vi "Query Heater Status.vi"(8 "error in (no error)":errorcluster, 10 "Output (0:Sample Heater)":u16(ring) items=["Sample Heater", "Warm-up Heater (Output 1)"], 11 "VISA resource name":refnum<visa-resource-name>) -> (0 "error out":errorcluster, 2 "Heater Status":u16(ring) items=["No Error (0)", "Heater Open Error (1)", "Heater Short Error (2)", "Voltage Compliance (3)"], 3 "VISA resource name out":refnum<visa-resource-name>)   [LabVIEW 2015, in "Lake Shore 372.lvlib"]
doc: "Queries if there is a heater open error.\n\nNote:\nThis only applies to sample heater and output 1 (warm-up heater)."
uses:
  <instrlib>/Lake Shore 372/Lake Shore 372.lvlib
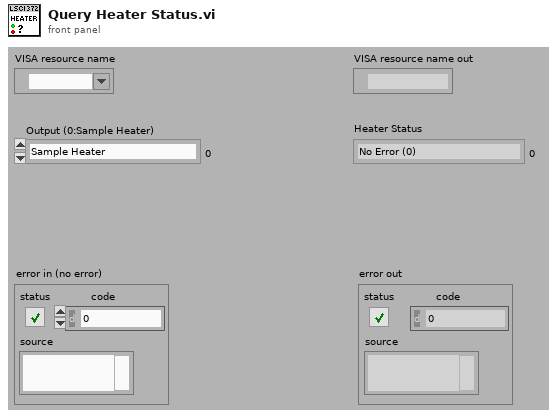
[diagram p1: front panel]
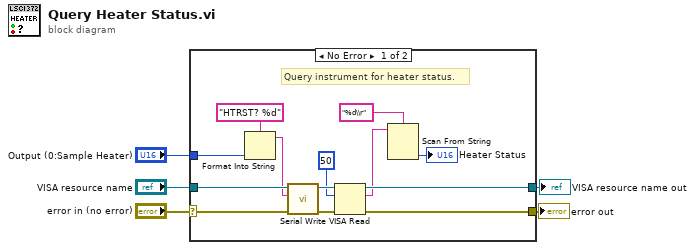
[diagram p0: block diagram]
diagram:
  n1 = case shown="No Error" "error in (no error)" {
    selector: "error in (no error)" -> [w6 w19]
    tunnel: [w18 w20] -> w5
    tunnel: [w17 w19] -> w4
    tunnel: "VISA resource name" -> [w16 w20]
    tunnel: "Output (0:Sample Heater)" -> [w10 _]
    frame No Error {
      # "Query instrument for heater status."
      n2 = Format Into String(format string="HTRST? %d", w10) -> (resulting string=w11:string)  [unwired: 2 in, 1 out]
      n3 = call <instrlib>:"Serial Write.vi"("error in (no error)"=w6, "Write Buffer (\"\")"=w11, "VISA resource name"=w16) -> ("error out"=w14:errorcluster, "VISA resource name out"=w15:refnum<visa-resource-name>)  [unwired: 6 in, 1 out]
      n4 = VISA Read(VISA resource name=w15, byte count=50, error in (no error)=w14) -> (VISA resource name out=w18:refnum<visa-resource-name>, read buffer=w8:string, error out=w17:errorcluster)  [unwired: 1 out]
      n5 = Scan From String(format string="%d\\r", input string=w8) -> (output 1=→"Heater Status":u16)  [unwired: 3 in, 3 out]
    }
    frame Error {
    }
  }
  "VISA resource name out" <- w5
  "error out" <- w4
